vi "MotorControl.vi"(9 "Stage Serial Number":i32=94839332, 11 "MG17Motor In":refnum<k7>) -> (3 "MG17Motor Out":refnum<k7>)   [LabVIEW 2012]
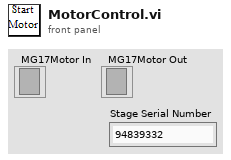
[diagram p1: front panel]
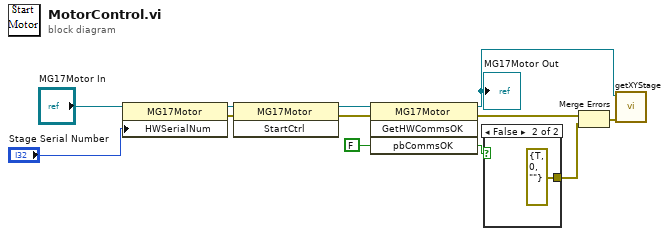
[diagram p0: block diagram]
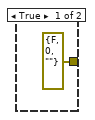
[diagram p2: hidden frame]
diagram:
  n1 = property class="MG17Motor"(reference="MG17Motor In", "HWSerialNum"="Stage Serial Number") -> (reference out=w3:refnum<k7>, error out=w2:errorcluster)  [unwired: 1 in]
  n2 = invoke class="MG17Motor" method="StartCtrl"(reference=w3, error in=w2) -> (reference out=w11:refnum<k7>, error out=w10:errorcluster)  [unwired: 1 in, 1 out]
  n3 = invoke class="MG17Motor" method="GetHWCommsOK"(reference=w11, error in=w10, "pbCommsOK"=FALSE) -> (reference out=w5:refnum<k7>, error out=w7:errorcluster, "pbCommsOK"=w8:bool)  [unwired: 1 in, 1 out]
  "MG17Motor Out" <- w5
  n4 = case shown="False" w8 {
    tunnel: [errorcluster {"status"=FALSE, "code"=0, "source"=""} ("error in (no error)") errorcluster {"status"=TRUE, "code"=0, "source"=""} ("error in (no error)")] -> w6
    frame True {
    }
    frame False {
    }
  }
  n5 = Merge Errors(w7, w6) -> (w4:errorcluster)
  n6 = call "getXYStage.vi"("error in (no error)"=w4, "Thorlabs APT Stage In"=w5) -> ()  [unwired: 9 in, 1 out]
